vi "remove_start_end_string.vi"(8 "error in (no error)":errorcluster, 9 "number of trailing characters to be removed":i32, 10 "number of leading characters to be removed":i32, 11 "input string":string) -> (0 "error out":errorcluster, 3 "output string":string)   [LabVIEW 2010]
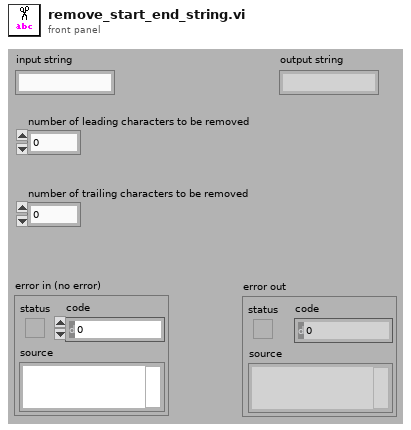
[diagram p1: front panel]
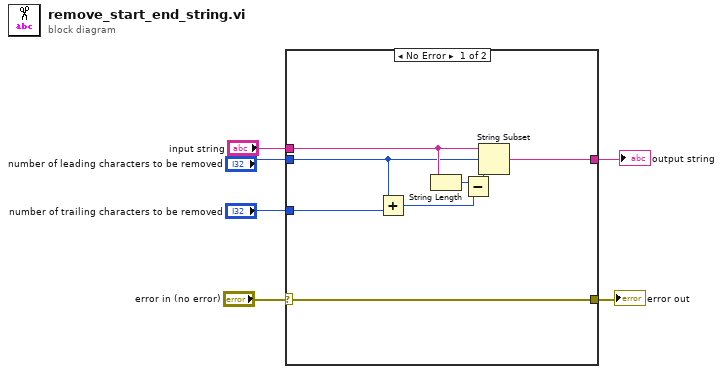
[diagram p0: block diagram]
diagram:
  n1 = case shown="No Error" "error in (no error)" {
    selector: "error in (no error)" -> [w11 w15]
    tunnel: "input string" -> [w10 w16]
    tunnel: [w12 w16] -> w5
    tunnel: [w11 w15] -> w3
    tunnel: "number of leading characters to be removed" -> [w9 _]
    tunnel: "number of trailing characters to be removed" -> [w8 _]
    frame No Error {
      n2 = Add(x=w9, y=w8) -> (x+y=w7:i32)
      n3 = String Length(string=w10) -> (length=w14:i32)
      n4 = Subtract(x=w14, y=w7) -> (x-y=w13:i32)
      n5 = String Subset(string=w10, offset (0)=w9, length (rest)=w13) -> (substring=w12:string)
    }
    frame Error {
    }
  }
  "error out" <- w3
  "output string" <- w5
